vi "Read Observables from string.vi"(11 "String":string) -> (0 "error in (no error)":errorcluster, 3 "Observables":T1[](array[typedef]) {"Weight" min=0.0 max=1.0})   [LabVIEW 2020, in "Run Utilities.lvlib" / "Optimiser Cell.lvclass"]
uses:
  Optimiser Cell.lvclass
  Optimisation observable.ctl
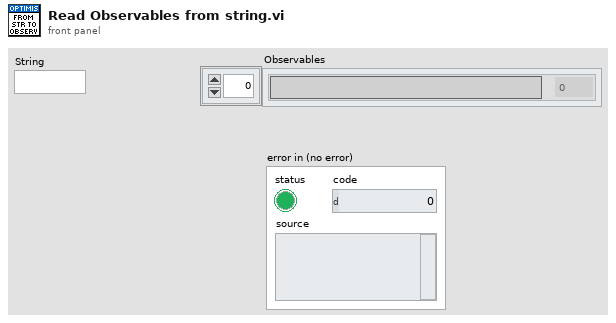
[diagram p1: front panel]
types:
  T1 = typedef "Run Utilities.lvlib/Optimiser Cell.lvclass/Optimisation observable.ctl" = cluster{"Name":string, "Weight":dbl}
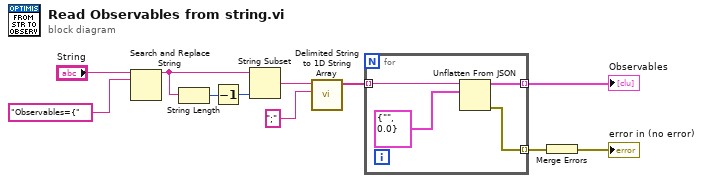
[diagram p0: block diagram]
diagram:
  n1 = Search and Replace String(input string="String", search string="Observables={") -> (result string=w9:string)  [unwired: 6 in, 3 out]
  n2 = String Length(string=w9) -> (length=w8:i32)
  n3 = Decrement(x=w8) -> (x-1=w7:i32)
  n4 = String Subset(string=w9, length (rest)=w7) -> (substring=w6:string)  [unwired: 1 in]
  n5 = call <vilib>:"Delimited String to 1D String Array.vi"("delimiter"=";", "delimited string"=w6) -> ("string array"=w4:string[])  [unwired: 9 in]
  n6 = for {
    tunnel: [w15] -> w1 mode=indexing
    tunnel: [w14] -> w3 mode=indexing
    tunnel: w4 -> [w13] mode=indexing
    n7 = Unflatten From JSON(JSON string=w13, type and defaults=T1 {"Name"="", "Weight"=0.0} ("Observable")) -> (value=w15:T1, error out=w14:errorcluster)  [unwired: 5 in]
  }
  "Observables" <- w1
  n8 = Merge Errors(w3) -> (→"error in (no error)":errorcluster)
